vi "MusicPlayer.vi"() -> ()   [LabVIEW 2019]
panel:
  out "Progress":u32(slide) scale=0.0..1000.0
  in  "Seek Forward Button":bool
  in  "Seek Back Button":bool
  in  "Media Stop Button":bool
  in  "Pause Button":bool
  in  "Play Button":bool
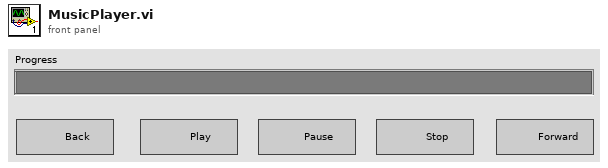
[diagram p1: front panel]
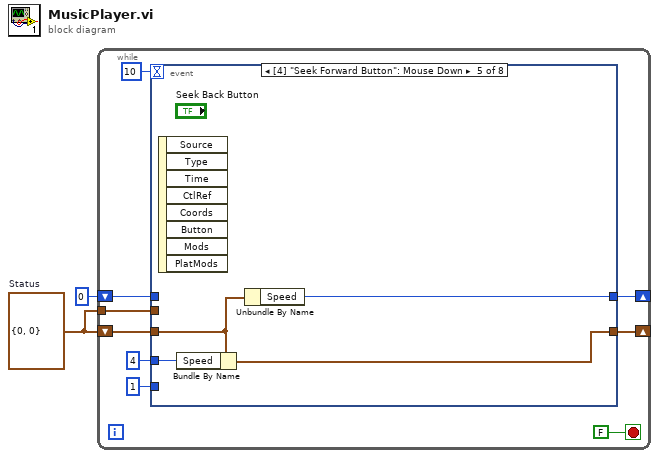
[diagram p0: block diagram]
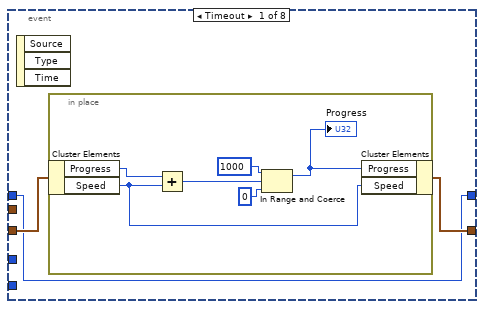
[diagram p2: hidden frame]
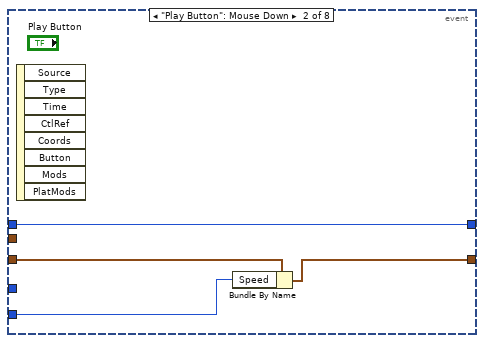
[diagram p3: hidden frame]
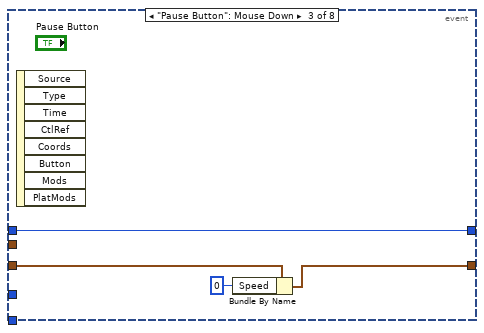
[diagram p4: hidden frame]
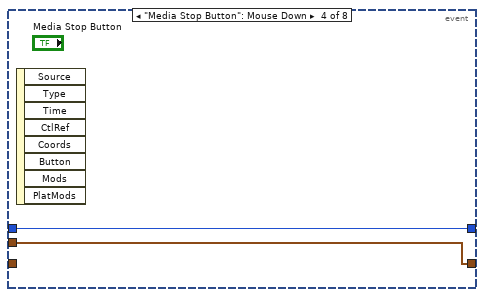
[diagram p5: hidden frame]
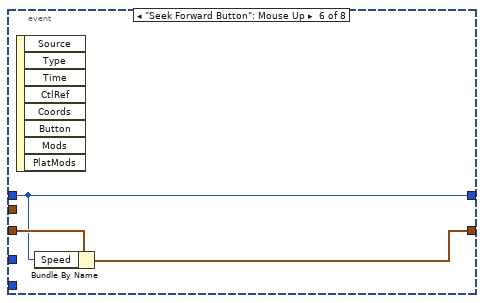
[diagram p6: hidden frame]
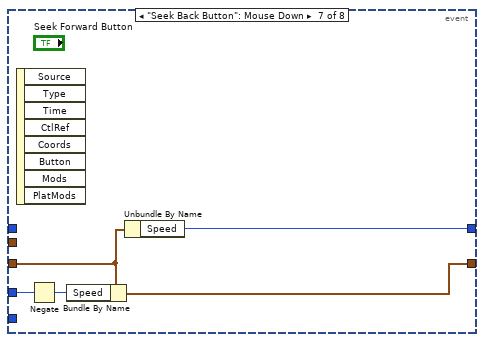
[diagram p7: hidden frame]
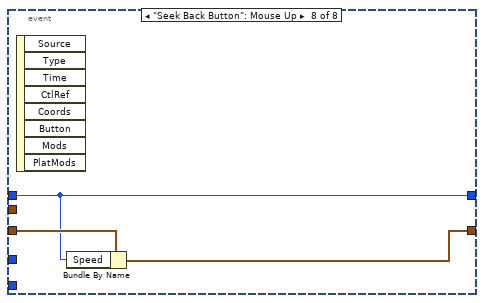
[diagram p8: hidden frame]
diagram:
  w2 = cluster{"Progress":i32, "Speed":i32} {"Progress"=0, "Speed"=0}  # Status
  n1 = while {
    shift-right: [w9] -> _
    shift-left: w2 -> [w10]
    tunnel: w2 -> [w7]
    shift-right: [w4] -> _
    shift-left: 0 ("Speed") -> [w3]
    stop <- FALSE stop-if-true
    n2 = event shown="[4] \"Seek Forward Button\": Mouse Down" {
      selector: _ -> [_ _ _ _ _ _ _ _]
      dyn-events: _ -> [_ _ _ _ _ _ _ _]
      timeout: 10 -> [_ _ _ _ _ _ _ _]
      tunnel: w10 -> [w14 w24 w28 _ w32 w37 w39 w45]
      tunnel: [w13 w23 w27 w30 w33 w36 w42 w44] -> w9
      tunnel: w7 -> [_ _ _ w30 _ _ _ _]
      tunnel: 4 ("Speed") -> [_ _ _ _ w34 _ w41 _]
      tunnel: 1 ("Speed") -> [_ w22 _ _ _ _ _ _]
      tunnel: [w12 w21 w25 w29 w31 w35 w38 w43] -> w4
      tunnel: w3 -> [w12 w21 w25 w29 _ w35 _ w43]
      event Timeout {
        n3 = event-data() -> ()  [unwired: 1 in, 3 out]
        n4 = in-place {
          n5 = in-place-cluster #1(w14) -> ("Progress"=w17:i32, "Speed"=w15:i32)
          n6 = Add(x=w17, y=w15) -> (x+y=w20:i32)
          n7 = In Range and Coerce(upper limit=1000, x=w20, lower limit=0 ("upper limit")) -> (coerced(x)=w16:i32)  [unwired: 1 out]
          "Progress" <- w16
          n8 = in-place-cluster #1("Progress"=w16, "Speed"=w15) -> (w13:cluster{"Progress":i32, "Speed":i32})
        }
      }
      event "Play Button": Mouse Down {
        n9 = event-data() -> ()  [unwired: 1 in, 8 out]
        n10 = Bundle By Name(cluster=w24, "Speed"=w22) -> (w23:cluster{"Progress":i32, "Speed":i32})
      }
      event "Pause Button": Mouse Down {
        n11 = event-data() -> ()  [unwired: 1 in, 8 out]
        n12 = Bundle By Name(cluster=w28, "Speed"=0) -> (w27:cluster{"Progress":i32, "Speed":i32})
      }
      event "Media Stop Button": Mouse Down {
        n13 = event-data() -> ()  [unwired: 1 in, 8 out]
      }
      event "Seek Forward Button": Mouse Down {
        n14 = event-data() -> ()  [unwired: 1 in, 8 out]
        n15 = Bundle By Name(cluster=w32, "Speed"=w34) -> (w33:cluster{"Progress":i32, "Speed":i32})
        n16 = Unbundle By Name(w32) -> ("Speed"=w31:i32)
      }
      event "Seek Forward Button": Mouse Up {
        n17 = event-data() -> ()  [unwired: 1 in, 8 out]
        n18 = Bundle By Name(cluster=w37, "Speed"=w35) -> (w36:cluster{"Progress":i32, "Speed":i32})
      }
      event "Seek Back Button": Mouse Down {
        n19 = event-data() -> ()  [unwired: 1 in, 8 out]
        n20 = Negate(x=w41) -> (-x=w40:i32)
        n21 = Bundle By Name(cluster=w39, "Speed"=w40) -> (w42:cluster{"Progress":i32, "Speed":i32})
        n22 = Unbundle By Name(w39) -> ("Speed"=w38:i32)
      }
      event "Seek Back Button": Mouse Up {
        n23 = event-data() -> ()  [unwired: 1 in, 8 out]
        n24 = Bundle By Name(cluster=w45, "Speed"=w43) -> (w44:cluster{"Progress":i32, "Speed":i32})
      }
    }
  }
